vi "Automation Hat Example.vi"() -> ()   [LabVIEW 2020]
doc: "An example showing the functionality of the Raspberry Pi Automation Hat LINX driver. Allows reading/writing from the various interfaces on the Automation Hat."
uses:
  LINX-AutomationHat/LEDs.ctl
  LINX-AutomationHat/DI Channels.ctl
  LINX-AutomationHat/ADC Channels.ctl
  <vilib>/MakerHub/LINX/Public/Utilities/Open Local.vi
  LINX-AutomationHat/LINX-AutomationHat.lvclass
  <vilib>/MakerHub/LINX/LMH-LINX.lvlib
panel:
  out "ADC Values":dbl[][](graph)
  out "ADC3":dbl format="%_3g"
  out "ADC2":dbl format="%_3g"
  out "ADC1":dbl format="%_3g"
  out "Input 3":bool
  out "Input 2":bool
  out "Input 1":bool
  in  "Auto LED Control":bool=TRUE
  in  "Output 3":bool
  in  "Output 2":bool
  in  "Output 1":bool
  out "Error Out":errorcluster
  in  "stop":bool
  in  "Warn":bool
  in  "Comms":bool
  in  "Power":bool
  in  "Relay 3":bool
  in  "Relay 2":bool
  in  "Relay 1":bool
  # "Raspberry Pi Automation Hat Example"
  # "This is a simple of example of using the AutomationHat LINX Addon driver for controlling the inputs/outputs of the Raspberry Pi LINX Automation Hat.\n\nIt had 3 0-24V ADCs, 3 sinking digital outputs, 3 buffered inputs, 3 relays and indicator LEDs."
  # "Enabling this will automatically control the LEDs according to the function."
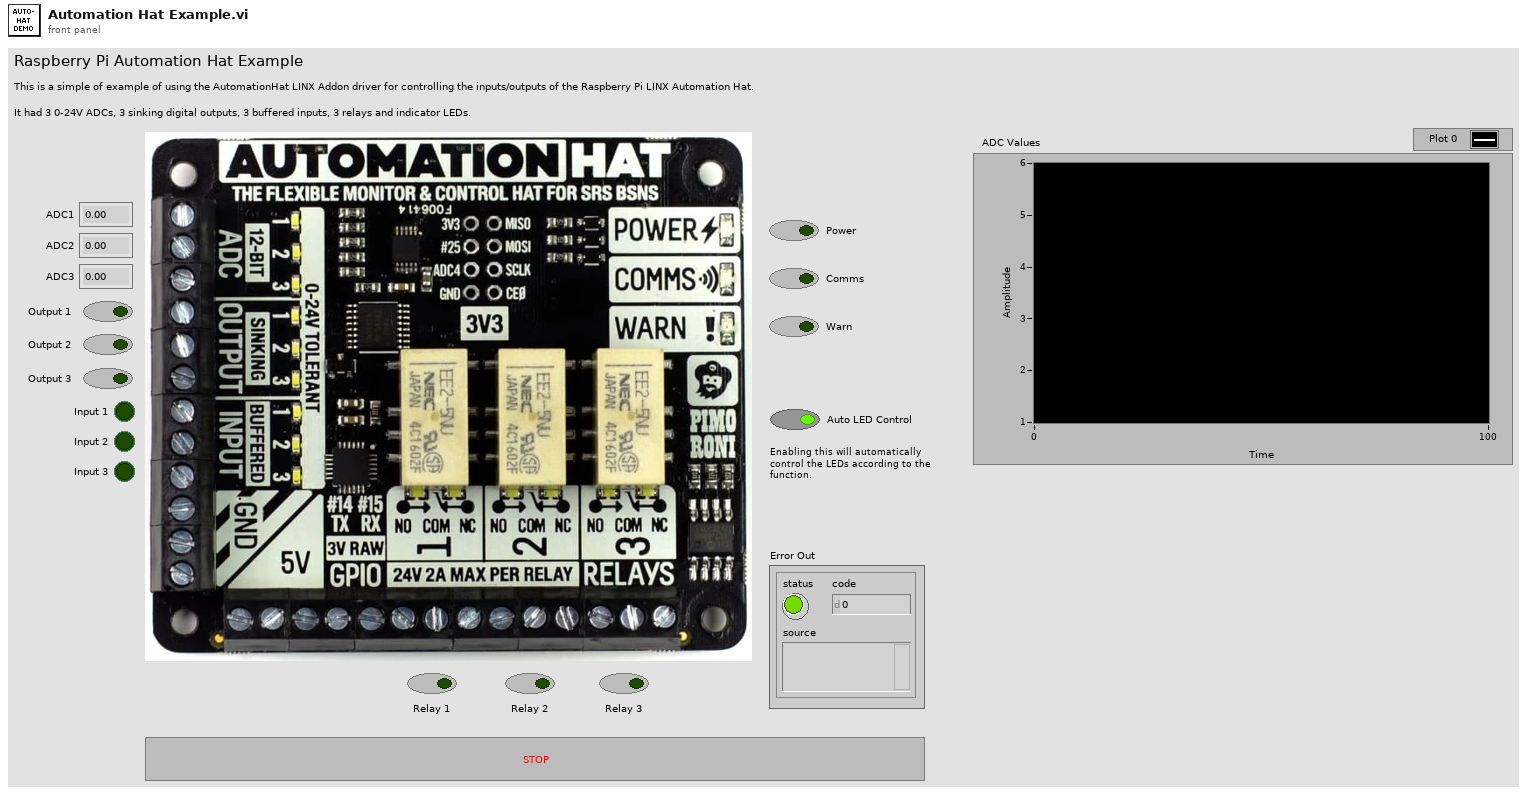
[diagram p1: front panel]
types:
  T1 = typedef "LMH-LINX.lvlib/LINX Ref.ctl" = cluster{"IO":T2, "Interface":T3, "LINX Device Config":T4}
  T2 = typedef "LMH-LINX.lvlib/Platform.ctl" = enum16{"Remote", "Local"}
  T3 = typedef "LMH-LINX.lvlib/Interface.ctl" = enum16{"Serial", "TCP"}
  T4 = typedef "LMH-LINX.lvlib/Device.lvlib/LINX Device Config.ctl" = cluster{"Interface":T3, "COM Port":refnum<visa-resource-name>, "TCP Configuration":T5, "Device Family":u8, "Device ID":u8, "Device Name":string, "TCP Ref":refnum<k5>, "Channels":T6}
  T5 = typedef "LMH-LINX.lvlib/Device.lvlib/TCP Config.ctl" = cluster{"IP Address":string, "Port":u16}
  T6 = typedef "LMH-LINX.lvlib/Channels.ctl" = cluster{"DI":u8[], "DO":u8[], "AI":u8[], "AO":u8[], "PWM":u8[], "QE":u8[], "UART":u8[], "I2C 2":u8[], "SPI":u8[], "CAN":u8[], "Servo":u8[], "AI Ref (V)":dbl, "AI Resolution (Bits)":u8, "AO Ref (V)":dbl, "AO Resolution (Bits)":u8}
  T7 = typedef "LINX-AutomationHat.lvclass/ADC Channels.ctl" = enum16{"ADC1 (24V)", "ADC2 (24V)", "ADC3 (24V)", "ADC4 (3.3v)"}
  T8 = typedef "LINX-AutomationHat.lvclass/DI Channels.ctl" = enum16{"Input1", "Input2", "Input3"}
  T9 = typedef "LINX-AutomationHat.lvclass/LEDs.ctl" = enum16{"All", "ADC1", "ADC2", "ADC3", "Output1", "Output2", "Output3", "Relay1NO", "Relay1NC", "Relay2NO", "Relay2NC", "Relay3NO", "Relay3NC", "Input3", "Input2", "Input1", "Warn", "Comms", "Power"}
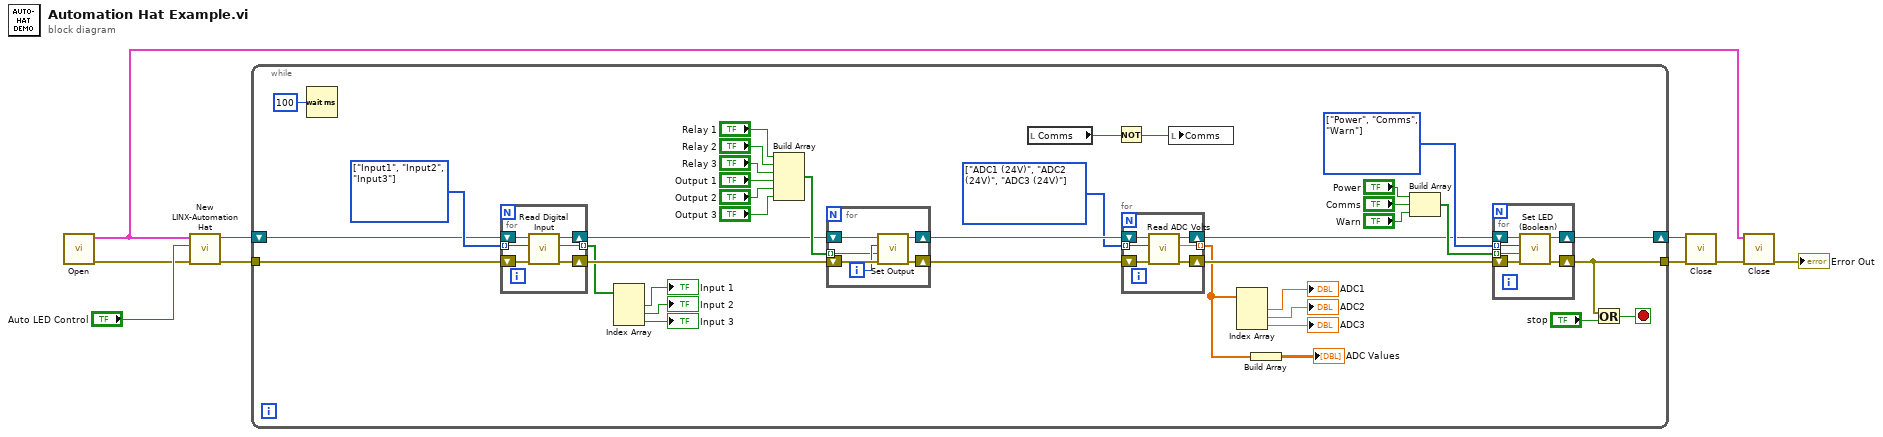
[diagram p0: block diagram]
diagram:
  n1 = call-poly <vilib>:"Open.vi"() -> ("Error Out"=w4:errorcluster, "LINX Resource"=w5:T1)  [unwired: 9 in, 1 out]
  n2 = call "New LINX-AutomationHat.vi"("error in (no error)"=w4, "Auto LED Control (T)"="Auto LED Control", "LINX Resource"=w5) -> ("error out"=w6:errorcluster, "LINX-AutomationHat out"=w7:refnum<class "LINX-AutomationHat.lvclass">)  [unwired: 7 in]
  n3 = while {
    tunnel: [w43] -> w2
    shift-right: [w44] -> w3
    shift-left: w7 -> [w29]
    tunnel: w6 -> [w28]
    stop <- w46 stop-if-true
    w17 = T7[] [enum."ADC1 (24V)", enum."ADC2 (24V)", enum."ADC3 (24V)"] items=["ADC1 (24V)", "ADC2 (24V)", "ADC3 (24V)", "ADC4 (3.3v)"] ("ADC Channel")
    w30 = T8[] [enum."Input1", enum."Input2", enum."Input3"] items=["Input1", "Input2", "Input3"] ("Input Channel")
    w42 = T9[] [enum."Power", enum."Comms", enum."Warn"] items=["All", "ADC1", "ADC2", "ADC3", "Output1", "Output2", "Output3", "Relay1NO", "Relay1NC", "Relay2NO", "Relay2NC", "Relay3NO", "Relay3NC", "Input3", "Input2", "Input1", "Warn", "Comms", "Power"] ("LED Selector")
    n4 = Wait (ms)(milliseconds to wait=u32 100) -> ()  [unwired: 1 out]
    n5 = for {
      tunnel: w30 -> [w59] mode=indexing
      shift-right: [w56] -> w27
      shift-left: w29 -> [w58]
      shift-right: [w55] -> w26
      shift-left: w28 -> [w57]
      tunnel: [w54] -> w25 mode=indexing
      n6 = call-dynamic "Read Digital Input.vi"("error in (no error)"=w57, "DI Channel"=w59, "LINX-AutomationHat in"=w58) -> ("error out"=w55:errorcluster, "Value"=w54:bool, "LINX-AutomationHat out"=w56:refnum<class "LINX-AutomationHat.lvclass">)  [unwired: 6 in]
    }
    n7 = Index Array(array=w25) -> (element #1=→"Input 1":bool, element #2=→"Input 2":bool, element #3=→"Input 3":bool)  [unwired: 3 in]
    n8 = Build Array("Relay 1", "Relay 2", "Relay 3", "Output 1", "Output 2", "Output 3") -> (w31:bool[])
    n9 = for {
      shift-right: [w64] -> w21
      shift-left: w27 -> [w65]
      shift-right: [w63] -> w20
      shift-left: w26 -> [w62]
      tunnel: w31 -> [w60] mode=indexing
      i -> [w61]
      n10 = call-dynamic "Set Output.vi"("error in (no error)"=w62, "Enable?"=w60, "Output Channel"=w61, "LINX-AutomationHat in"=w65) -> ("error out"=w63:errorcluster, "LINX-AutomationHat out"=w64:refnum<class "LINX-AutomationHat.lvclass">)  [unwired: 6 in]
    }
    n11 = local read "Comms"() -> (w13:bool)
    n12 = Not(x=w13) -> (.not. x?=w12:bool)
    n13 = for {
      tunnel: w17 -> [w49] mode=indexing
      shift-right: [w51] -> w19
      shift-left: w21 -> [w53]
      shift-right: [w50] -> w18
      shift-left: w20 -> [w52]
      tunnel: [w48] -> w11 mode=indexing
      n14 = call-dynamic "Read ADC Volts.vi"("error in (no error)"=w52, "ADC Channel"=w49, "LINX-AutomationHat in"=w53) -> ("error out"=w50:errorcluster, "Value (V)"=w48:dbl, "LINX-AutomationHat out"=w51:refnum<class "LINX-AutomationHat.lvclass">)  [unwired: 6 in]
    }
    n15 = local write "Comms"(w12) -> ()
    n16 = Index Array(array=w11) -> (element #1=→"ADC1":dbl, element #2=→"ADC2":dbl, element #3=→"ADC3":dbl)  [unwired: 3 in]
    n17 = Build Array(w11) -> (→"ADC Values":dbl[][])
    n18 = Build Array("Power", "Comms", "Warn") -> (w38:bool[])
    n19 = for {
      shift-right: [w70] -> w44
      shift-left: w19 -> [w71]
      shift-right: [w69] -> w43
      shift-left: w18 -> [w68]
      tunnel: w42 -> [w67] mode=indexing
      tunnel: w38 -> [w66] mode=indexing
      n20 = call-dynamic "Set LED (Boolean).vi"("error in (no error)"=w68, "Enable"=w66, "LED Selector"=w67, "LINX-AutomationHat in"=w71) -> ("error out"=w69:errorcluster, "LINX-AutomationHat out"=w70:refnum<class "LINX-AutomationHat.lvclass">)  [unwired: 6 in]
    }
    n21 = Or(x=w43, y="stop") -> (x .or. y?=w46:bool)
  }
  n22 = call-dynamic <vilib>:"Close.vi"("error in (no error)"=w2, "LINX-AutomationHat in"=w3) -> ("error out"=w1:errorcluster)  [unwired: 8 in, 1 out]
  n23 = call <vilib>:"Close.vi"("Error In"=w1, "LINX Resource"=w5) -> ("Error Out"=→"Error Out":errorcluster)  [unwired: 9 in]
